vi "GetClassPathfromIDNStrPath.vi"(8 "error in (no error)":errorcluster, 11 "Path in":path) -> (0 "error out":errorcluster, 3 "Path out":path)   [LabVIEW 2014]
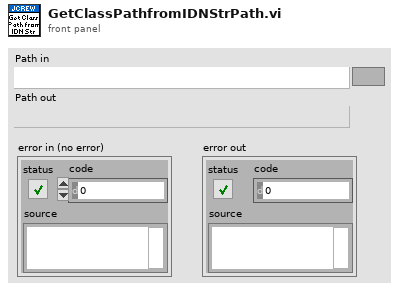
[diagram p1: front panel]
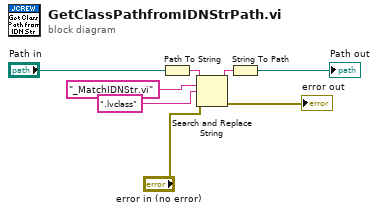
[diagram p0: block diagram]
diagram:
  n1 = Path To String(path="Path in") -> (string=w5:string)
  n2 = Search and Replace String(input string=w5, search string="_MatchIDNStr.vi" ("regular expression"), replace string=".lvclass" ("pattern"), error in="error in (no error)") -> (result string=w8:string, error out=→"error out":errorcluster)  [unwired: 4 in, 2 out]
  n3 = String To Path(string=w8) -> (path=→"Path out":path)
